vi "Upsample.vi"(8 "error in":errorcluster, 10 "inputData":cdb[](array[numeric]), 11 "Path In":path) -> (0 "error out":errorcluster, 2 "out_data":cdb[](array[numeric]), 3 "Path Out":path)   [LabVIEW 2015]
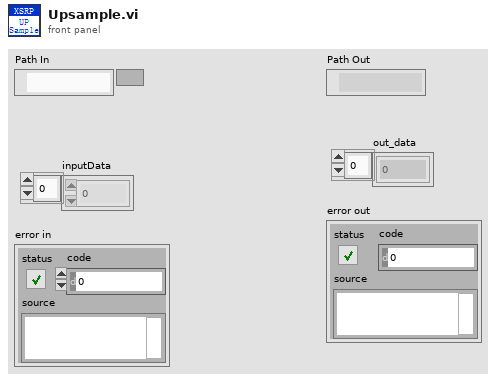
[diagram p1: front panel]
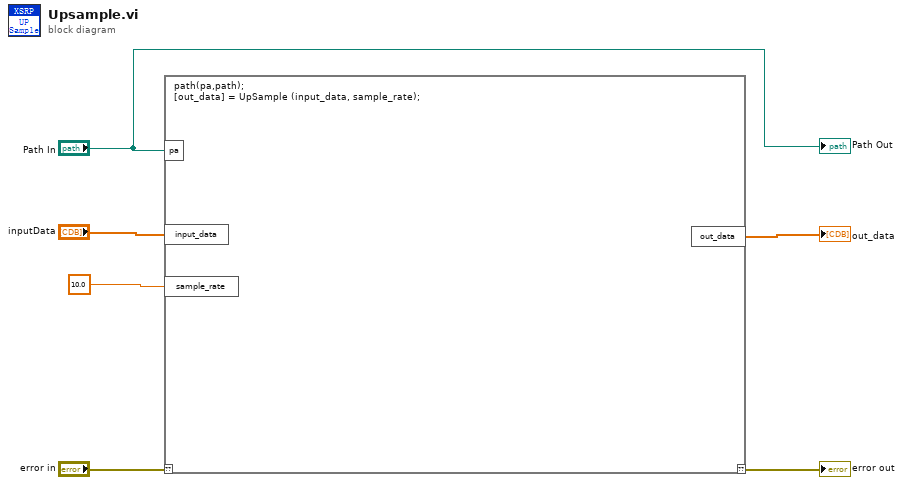
[diagram p0: block diagram]
diagram:
  n1 = script code="path(pa,path);\n[out_data] = UpSample (input_data, sample_rate);"("??"="error in", "pa"="Path In", "input_data"="inputData", "sample_rate"=10.0) -> ("??"=→"error out":errorcluster, "out_data"=→"out_data":cdb[])
  "Path Out" <- "Path In"
